vi "dfd_DFXP_Right Shift (scaler).vi"(9 "High 64":i64, 10 "Low 64":u64, 11 "Num":i16) -> (1 "High 64":i64, 2 "Low 64":u64)   [LabVIEW 2017, in "NI_DigFilter_FXP.lvlib"]
uses:
  <vilib>/addons/Digital Filter Design/NI_DigFilter_FXP.lvlib
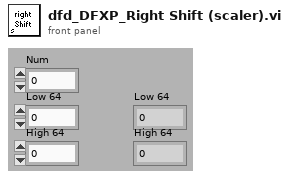
[diagram p1: front panel]
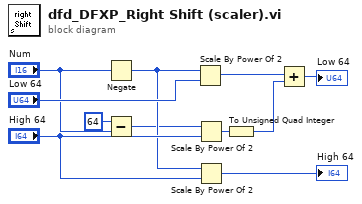
[diagram p0: block diagram]
diagram:
  n1 = Negate(x="Num") -> (-x=w4:i16)
  n2 = Subtract(x=i16 64 ("y"), y="Num") -> (x-y=w3:i16)
  n3 = Scale By Power Of 2(n=w4, x="Low 64") -> (x*2^n=w5:u64)
  n4 = Scale By Power Of 2(n=w3, x="High 64") -> (x*2^n=w2:i64)
  n5 = Scale By Power Of 2(n=w4, x="High 64") -> (x*2^n=→"High 64":i64)
  n6 = To Unsigned Quad Integer(1:w2) -> (0:w1:u64)
  n7 = Add(x=w5, y=w1) -> (x+y=→"Low 64":u64)
